vi "Look up Available Measurement by Name.vi"(8 "error in (no error)":errorcluster, 10 "Measurement Name":string, 11 "Mag Lab Measure Controller in":refnum<class "Mag Lab Measure Controller.lvclass">) -> (0 "error out":errorcluster, 2 "Measurement queue":refnum<class "Message Enqueuer.lvclass">, 3 "Mag Lab Measure Controller out":refnum<class "Mag Lab Measure Controller.lvclass">)   [LabVIEW 2015, in "Mag Lab Measure Controller.lvclass"]
uses:
  Mag Lab Measure Controller.lvclass
  <vilib>/ActorFramework/Message Enqueuer/Message Enqueuer.lvclass
  Mag Lab Measure Controller.lvclass/Mag Lab Measure Controller.ctl
  Mag Lab Error Handler/Mag Lab Error Handler.lvclass
panel:
  out "found":bool
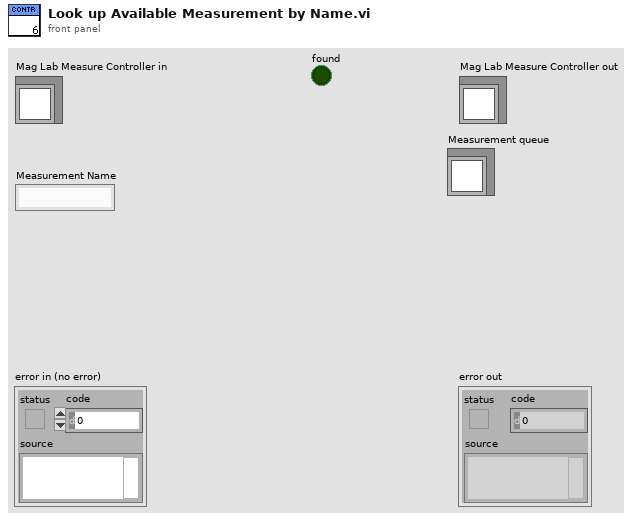
[diagram p1: front panel]
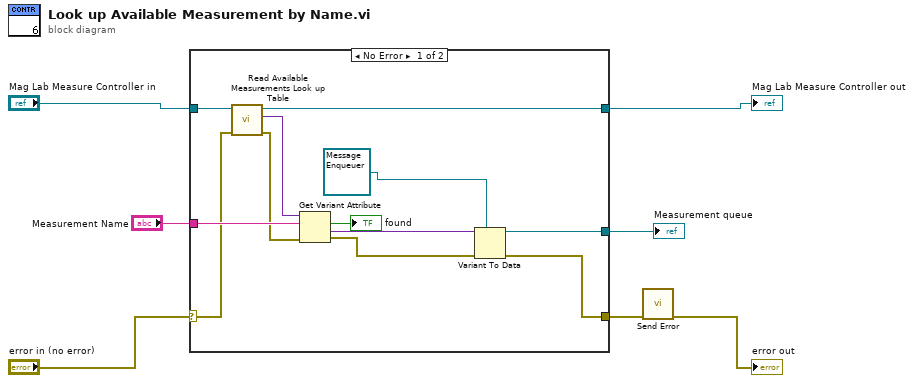
[diagram p0: block diagram]
diagram:
  n1 = case shown="No Error" "error in (no error)" {
    selector: "error in (no error)" -> [w11 w21]
    tunnel: [w10 w21] -> w2
    tunnel: [w17 w20] -> w5
    tunnel: "Mag Lab Measure Controller in" -> [w19 w20]
    tunnel: "Measurement Name" -> [w16 _]
    tunnel: [w14 _] -> w3
    frame No Error {
      n2 = call "Read Available Measurements Look up Table.vi"("error in (no error)"=w11, "Mag Lab Measure Controller in"=w19) -> ("error out"=w13:errorcluster, "Available Measurement Objects Lookup Table (Msmt Name -> Measurement.lvclass)"=w18:variant, "Mag Lab Measure Controller out"=w17:refnum<class "Mag Lab Measure Controller.lvclass">)  [unwired: 7 in]
      n3 = Get Variant Attribute(Variant=w18, name=w16, error in=w13) -> (found=→"found":bool, value=w15:variant, error out=w12:errorcluster)  [unwired: 1 in, 1 out]
      n4 = Variant To Data(error in=w12, type=refnum<class "Message Enqueuer.lvclass"> refnum ("Self Enqueuer"), Variant=w15) -> (data=w14:refnum<class "Message Enqueuer.lvclass">, error out=w10:errorcluster)
    }
    frame Error {
    }
  }
  "Mag Lab Measure Controller out" <- w5
  "Measurement queue" <- w3
  n5 = call "Send Error.vi"("error in (no error)"=w2) -> ("error out"=→"error out":errorcluster)  [unwired: 9 in, 1 out]
